vi "ZmParam_PH.vi"() -> ()   [LabVIEW 2021]
panel:
  in  "stop":bool
  out "Waveform Chart":dbl(graph)=0.0896154250709622
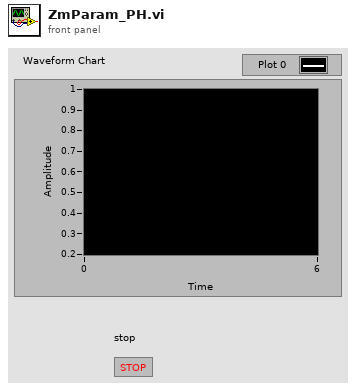
[diagram p1: front panel]
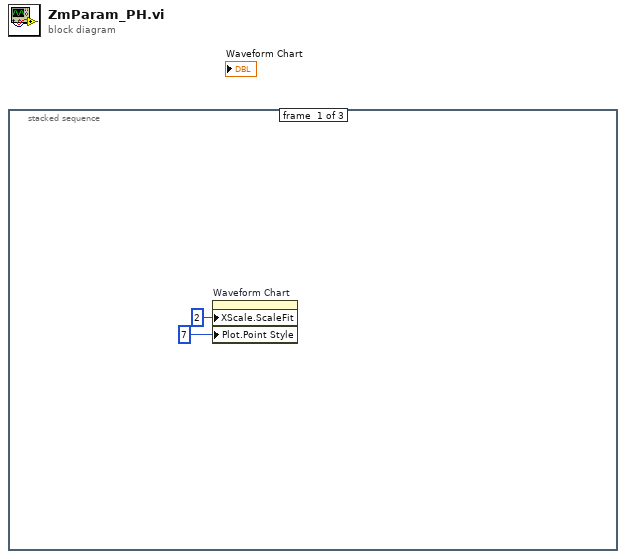
[diagram p0: block diagram]
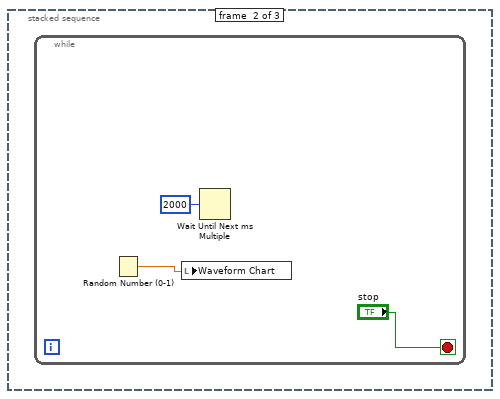
[diagram p2: hidden frame]
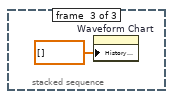
[diagram p3: hidden frame]
diagram:
  n1 = stacked-sequence {
    frame #0 {
      n2 = property on="Waveform Chart" class="WFChart (strict)"("XScale.ScaleFit"=u8 2 ("X Scale.Scale Fit"), "Plot.Point Style"=u8 7) -> ()  [unwired: 2 in, 2 out]
    }
    frame #1 {
      n3 = while {
        stop <- "stop" stop-if-true
        n4 = Random Number (0-1)() -> (number: 0 to 1=w4:dbl)
        n5 = local write "Waveform Chart"(w4) -> ()
        n6 = Wait Until Next ms Multiple(millisecond multiple=u32 2000) -> ()  [unwired: 1 out]
      }
    }
    frame #2 {
      n7 = property on="Waveform Chart" class="WFChart (strict)"("History Data"=dbl[] []) -> ()  [unwired: 2 in, 2 out]
    }
  }
